vi "Drive.vi"(7 "Slow?":bool, 9 "SwitchDir":bool=TRUE, 10 "Drive L":dbl, 11 "Drive R":dbl) -> ()   [LabVIEW 2016]
panel:
  in  "Drive Reduction":dbl=0.4 format="%#_13g"
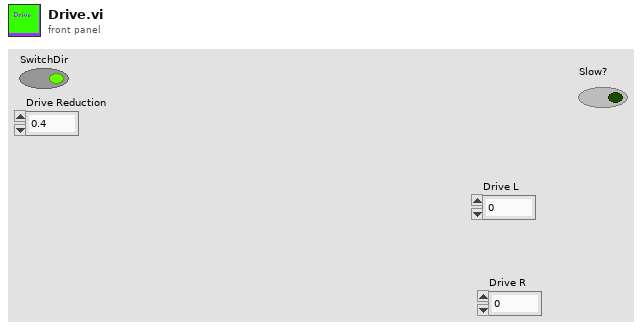
[diagram p1: front panel]
types:
  T1 = typedef "WPI_MotorControlDeviceRef.ctl" = cluster{"DeviceStatus":errorcluster, "Type":T2, "PWM":cluster{"PWM Channel":T3, "DeadBand":T4}, "CAN":cluster{"Device Number":u8, "SetOutput VI Ref":variant, "GetOutput VI Ref":variant, "Enable VI Ref":variant, "Disable VI Ref":variant, "Data":variant}, "Invert":bool}
  T2 = typedef "WPI_MotorControlType.ctl" = enum16{"PWM", "CAN"}
  T3 = typedef "FPGA_DIOPWMChannel.ctl" = enum8{"PWM 0", "PWM 1", "PWM 2", "PWM 3", "PWM 4", "PWM 5", "PWM 6", "PWM 7", "PWM 8", "PWM 9", "PWM MXP 0", "PWM MXP 1", "PWM MXP 2", "PWM MXP 3", "PWM MXP 4", "PWM MXP 5", "PWM MXP 6", "PWM MXP 7", "PWM MXP 8", "PWM MXP 9", "Invalid"}
  T4 = typedef "WPI_PWMDeadband.ctl" = cluster{"Name":string, "maxPositivePwm":i32, "minPositivePwm":i32, "centerPwm":i32, "maxNegativePwm":i32, "minNegativePwm":i32, "angularRange":u16}
  T5 = typedef "WPI_CANTalonSRX_GlobalStatus.ctl" = cluster{"Applied Throttle":dbl, "Module Enabled":bool, "CAN Error":errorcluster, "Closed Loop Error":dbl, "Forward Limit Switch Closed":bool, "Reverse Limit Switch Closed":bool, "Sensor Position":dbl, "Sensor Velocity":dbl, "Current":dbl, "Sticky Fault - Over Temp":bool, "Sticky Fault - Under Voltage":bool, "Sticky Fault - Forward Limit":bool, "Sticky Fault - Reverse Limit":bool, "Sticky Fault - Forward Soft Limit":bool, "Sticky Fault - Reverse Soft Limit":bool, "Brake is Enabled":bool, "Encoder Position":dbl, "Encoder Velocity":dbl, "Encoder Index Count":dbl, "Encoder A Pin State":bool, "Encoder B Pin State":bool, "Encoder Index Pin State":bool, "Analog In":dbl, "Analog In Velocity":dbl, "Temperature (C)":dbl, "Battery Voltage":dbl, "Control 5 Is Supported":bool, "Current Profile Slot Select":dbl, "Pos Div 8":bool, "Vel Div 4":bool, "Pulse Width Position":i32, "Pulse Width Velocity":i32, "Pulse Width Rise To Rise (us)":i32, "Pulse Width Rise To Fall (us)":i32, "Mot Prof Active Is Under Run":bool, "Mot Prof Active Has Under Run":bool, "Mot Prof Active Is Last":bool, "Mot Prof Active Velocity Only":bool, "Mot Prof Active Is Valid":bool, "Mot Prof Buffer Is Full":bool, "Mot Prof Active Profile Slot Select":i32, "Mot Prof NextID":i32, "Mot Prof Count":i32, "Mot Prof Active Velocity":dbl, "Mot Prof Active Position":dbl, "Mot Prof Output Enable":i32}
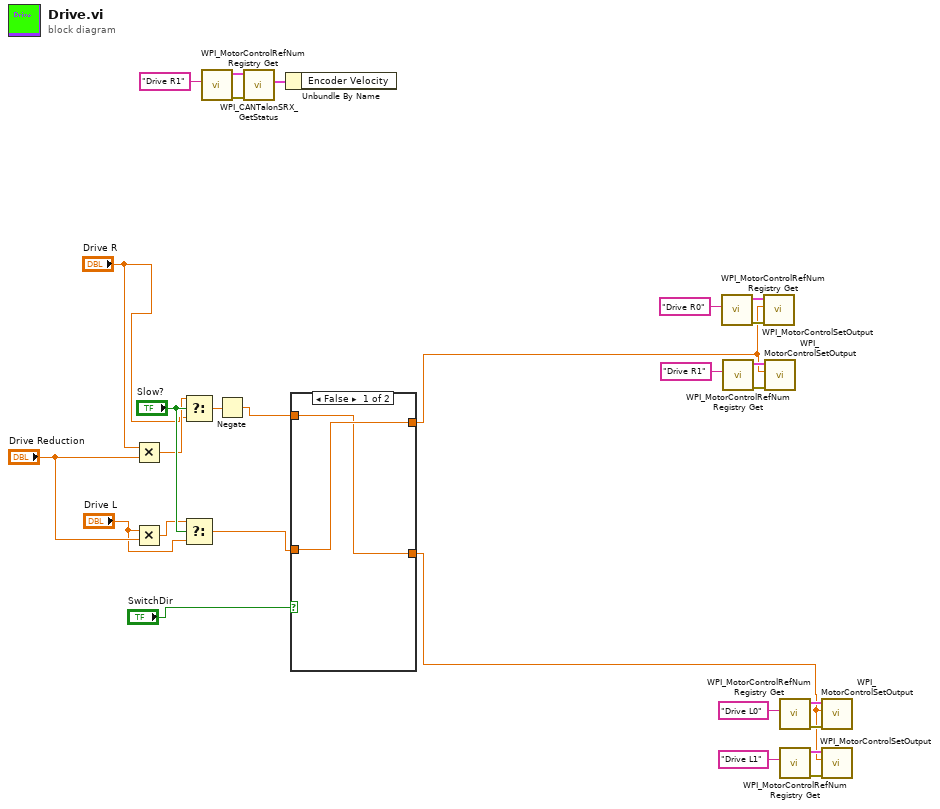
[diagram p0: block diagram]
diagram:
  n1 = Multiply(x="Drive R", y="Drive Reduction") -> (x*y=w10:dbl)
  n2 = Multiply(x="Drive L", y="Drive Reduction") -> (x*y=w8:dbl)
  n3 = Select(t=w10, s="Slow?", f="Drive R") -> (s? t:f=w15:dbl)
  n4 = Select(t=w8, s="Slow?", f="Drive L") -> (s? t:f=w13:dbl)
  n5 = call <vilib>:"WPI_MotorControlRefNum Registry Get.vi"("refnum name"="Drive R1") -> ("error out"=w5:errorcluster, "MotorControlDevRef"=w6:T1)  [unwired: 9 in]
  n6 = Negate(x=w15) -> (-x=w14:dbl)
  n7 = call <vilib>:"WPI_CANTalonSRX_GetStatus.vi"("error in (no error)"=w5, "CAN Talon SRX Ref"=w6) -> ("Talon SRX Status"=w4:T5)  [unwired: 7 in, 2 out]
  n8 = Unbundle By Name(w4) -> ()  [unwired: 1 out]
  n9 = case shown="False" "SwitchDir" {
    tunnel: [w30 w31] -> w1
    tunnel: w14 -> [w29 w32]
    tunnel: [w29 w32] -> w2
    tunnel: w13 -> [w30 w31]
    frame False {
    }
    frame True {
    }
  }
  n10 = call <vilib>:"WPI_MotorControlRefNum Registry Get.vi"("refnum name"="Drive R0") -> ("error out"=w22:errorcluster, "MotorControlDevRef"=w18:T1)  [unwired: 9 in]
  n11 = call <vilib>:"WPI_MotorControlRefNum Registry Get.vi"("refnum name"="Drive R1") -> ("error out"=w17:errorcluster, "MotorControlDevRef"=w20:T1)  [unwired: 9 in]
  n12 = call <vilib>:"WPI_MotorControlSetOutput.vi"("error in (no error)"=w22, "Output"=w1, "MotorControlDevRef"=w18) -> ()  [unwired: 6 in, 3 out]
  n13 = call <vilib>:"WPI_MotorControlSetOutput.vi"("error in (no error)"=w17, "Output"=w1, "MotorControlDevRef"=w20) -> ()  [unwired: 6 in, 3 out]
  n14 = call <vilib>:"WPI_MotorControlRefNum Registry Get.vi"("refnum name"="Drive L0") -> ("error out"=w23:errorcluster, "MotorControlDevRef"=w24:T1)  [unwired: 9 in]
  n15 = call <vilib>:"WPI_MotorControlRefNum Registry Get.vi"("refnum name"="Drive L1") -> ("error out"=w27:errorcluster, "MotorControlDevRef"=w26:T1)  [unwired: 9 in]
  n16 = call <vilib>:"WPI_MotorControlSetOutput.vi"("error in (no error)"=w23, "Output"=w2, "MotorControlDevRef"=w24) -> ()  [unwired: 6 in, 3 out]
  n17 = call <vilib>:"WPI_MotorControlSetOutput.vi"("error in (no error)"=w27, "Output"=w2, "MotorControlDevRef"=w26) -> ()  [unwired: 6 in, 3 out]
